vi "RT Loop - Stage Position Monitoring.vi"(11 "VISA resource name":refnum<visa-resource-name>) -> ()   [LabVIEW 2013]
uses:
  Globals/Global - Configuration Options.vi
  Globals/Global - All RT Loop Stop.vi
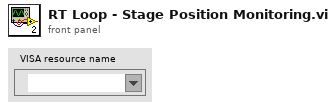
[diagram p1: front panel]
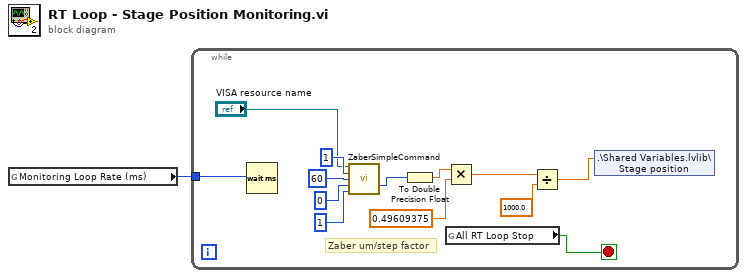
[diagram p0: block diagram]
diagram:
  n1 = global read "Global - Configuration Options.vi" "Monitoring Loop Rate (ms)"() -> (w1:u32)
  n2 = while {
    tunnel: w1 -> [w7]
    stop <- w8 stop-if-true
    # "Zaber um/step factor"
    n3 = Wait (ms)(milliseconds to wait=w7) -> ()  [unwired: 1 out]
    n4 = call "ZaberSimpleCommand.vi"("VISA Refnum in"="VISA resource name", "Num1"=1, "Cmd"=60, "Val"=0, "Resp num"=1) -> ("Val"=w10:i32)  [unwired: 8 in, 2 out]
    n5 = To Double Precision Float(number=w10) -> (double precision float=w3:dbl)
    n6 = Multiply(x=w3, y=0.49609375) -> (x*y=w6:dbl)
    n7 = global read "Global - All RT Loop Stop.vi" "All RT Loop Stop"() -> (w8:bool)
    n8 = Divide(x=w6, y=1000.0) -> (x/y=w4:dbl)
    n9 = shared-variable ".\\Shared Variables.lvlib\\Stage position"(w4) -> ()  [unwired: 1 in, 1 out]
  }
